vi "Get System Channel Properties.vi"(8 "error in (no error)":errorcluster, 10 "System Channel Refnums":T1[](array[typedef]) format="%.0x", 11 "Device Reference in":T1 format="%.0x") -> (0 "error out":errorcluster, 2 "System Channel Properties":T2, 3 "Device Reference out":T1=18446744073709551615 format="%.0x")   [LabVIEW 2019, in "Telemetry Engine.lvlib"]
doc: "This VI reads the necessary Log File Properties like: Channel Names, Channel Properties and other."
uses:
  Telemetry Engine.lvlib
  <vilib>/NI VeriStand/Custom Device API/Custom Device Item Ref.ctl
  Types/System Channels.ctl
  Shared/Constants.vi
  <vilib>/NI VeriStand/Custom Device API/Custom Device API.lvlib
  Shared/Telemetry Shared.lvlib
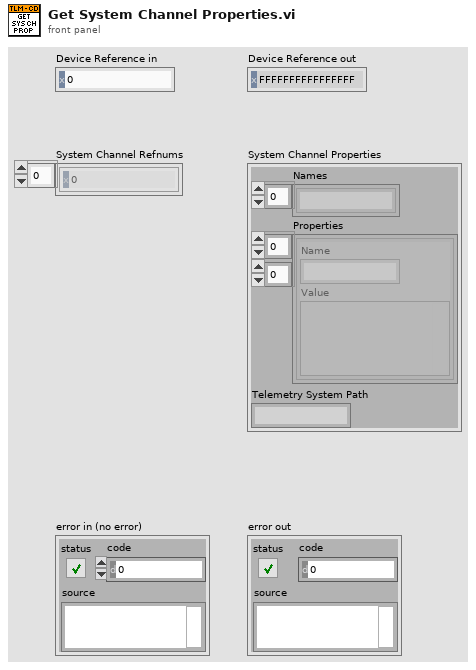
[diagram p1: front panel]
types:
  T1 = typedef "Custom Device API.lvlib/Custom Device Item Ref.ctl" = u64
  T2 = typedef "Telemetry Engine.lvlib/System Channels.ctl" = cluster{"Names":string[], "Properties":cluster{"Name":string, "Value":variant}[][], "Telemetry System Path":string}
  T3 = typedef "Custom Device API.lvlib/Custom Device Item Info.ctl" = cluster{"Name":string, "Is Channel":bool, "GUID":string, "Is Waveform":bool}
  T4 = cluster{"Description":string, "Variant":variant}[]
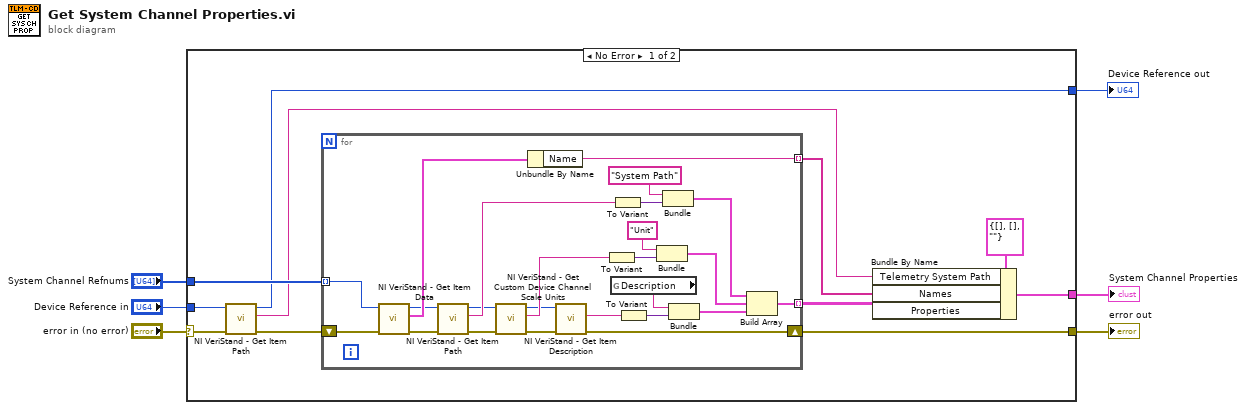
[diagram p0: block diagram]
diagram:
  n1 = case shown="No Error" "error in (no error)" {
    selector: "error in (no error)" -> [w9 w43]
    tunnel: "Device Reference in" -> [w11 w42]
    tunnel: [w17 w43] -> w5
    tunnel: "System Channel Refnums" -> [w16 _]
    tunnel: [w12 _] -> w2
    tunnel: [w7 w42] -> w1
    frame No Error {
      n2 = call <vilib>:"NI VeriStand - Get Item Path.vi"("error in (no error)"=w9, "Item Ref in"=w11) -> ("error out"=w8:errorcluster, "Path"=w10:string, "Item Ref out"=w7:T1)  [unwired: 6 in, 1 out]
      n3 = for {
        tunnel: w16 -> [w40] mode=indexing
        shift-right: [w39] -> w17
        shift-left: w8 -> [w29]
        tunnel: [w38] -> w13 mode=indexing
        tunnel: [w19] -> w15 mode=indexing
        n4 = call <vilib>:"NI VeriStand - Get Item Data.vi"("error in (no error)"=w29, "Item Ref in"=w40) -> ("error out"=w34:errorcluster, "Item Info"=w41:T3, "Item Ref out"=w28:T1)  [unwired: 6 in, 1 out]
        n5 = call <vilib>:"NI VeriStand - Get Item Path.vi"("error in (no error)"=w34, "Item Ref in"=w28) -> ("error out"=w27:errorcluster, "Path"=w31:string, "Item Ref out"=w25:T1)  [unwired: 6 in, 1 out]
        n6 = call <vilib>:"NI VeriStand - Get Custom Device Channel Scale Units.vi"("error in (no error)"=w27, "Channel Ref in"=w25) -> ("error out"=w26:errorcluster, "ScaleUnits"=w22:string, "Channel Ref out"=w21:T1)  [unwired: 7 in]
        n7 = Unbundle By Name(w41) -> ("Name"=w38:string)
        n8 = call <vilib>:"NI VeriStand - Get Item Description.vi"("error in (no error)"=w26, "Item Ref in"=w21) -> ("error out"=w39:errorcluster, "Description"=w37:string)  [unwired: 6 in, 2 out]
        n9 = To Variant(anything=w22) -> (Variant=w24:variant)
        n10 = global read "Constants.vi" "Description"() -> (w18:string)
        n11 = To Variant(anything=w31) -> (Variant=w32:variant)
        n12 = To Variant(anything=w37) -> (Variant=w36:variant)
        n13 = Bundle("Description"="Unit", "Variant"=w24) -> (w20:cluster{"Description":string, "Variant":variant})  [unwired: 1 in]
        n14 = Bundle("Description"="System Path", "Variant"=w32) -> (w30:cluster{"Description":string, "Variant":variant})  [unwired: 1 in]
        n15 = Bundle("Description"=w18, "Variant"=w36) -> (w35:cluster{"Description":string, "Variant":variant})  [unwired: 1 in]
        n16 = Build Array(w30, w20, w35) -> (w19:T4)
      }
      n17 = Bundle By Name(cluster=T2 {"Names"=[], "Properties"=[], "Telemetry System Path"=""} ("input cluster"), "Telemetry System Path"=w10, "Names"=w13, "Properties"=w15) -> (w12:T2)
    }
    frame Error {
    }
  }
  "error out" <- w5
  "System Channel Properties" <- w2
  "Device Reference out" <- w1
